vi "clearpath_set_max_speed.vi"(0 "ClearpathComm":T1, 1 "Max Speed":dbl) -> ()   [LabVIEW 2012, in "clearpath_interface.lvlib"]
doc: "Formats a Set Max Speed command (0x210) to change the built-in maximum speed (in m/s). Can not be set to a value greater than the factory default, but can be set lower. Resetting the processor or power cycling the platform will reset the setting to default. Uses the onboard Clearpath library to perform the actual message formatting."
uses:
  clearpath_interface.lvlib
  cwrap_crio.dll
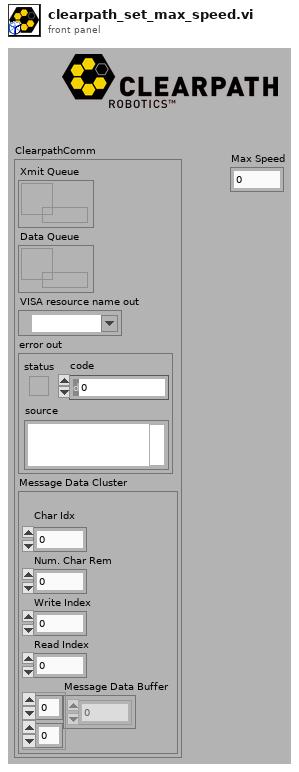
[diagram p1: front panel]
types:
  T1 = cluster{"Xmit Queue":refnum<queue>, "Data Queue":refnum<queue>, "VISA resource name out":refnum<visa-resource-name>, "error out":errorcluster, "Message Data Cluster":cluster{"\nChar Idx":u8, "Num. Char Rem":u8, "Write Index":u8, "Read Index":u8, "Message Data Buffer":u8[][]}}
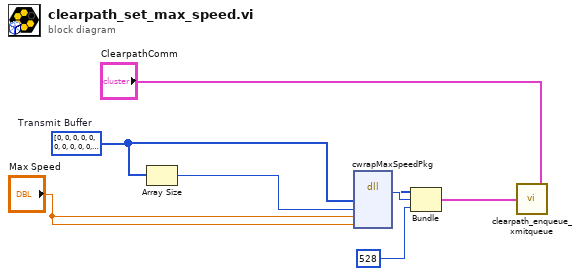
[diagram p0: block diagram]
diagram:
  w5 = u8[] [0, 0, 0, 0, 0, 0, 0, 0, 0, 0, 0, 0, 0, 0, 0, 0, 0, 0, 0, 0, 0, 0, 0, 0, 0, 0, 0, 0, 0, 0, 1, 0, 0, 0, 5]  # Transmit Buffer
  n1 = Array Size(array=w5) -> (size(s)=w6:i32)
  n2 = dll-call lib="C:/Users/tebbeam/Documents/GitHub/IGVC-2013/Code/Project 1.0/Motors/Husky/cwrap_cRIO.*" fn="cwrapMaxSpeedPkg"("buf"=w5, "buf_size"=w6, "max_fwd"="Max Speed", "max_rev"="Max Speed") -> ("return type"=w8:i32, "buf"=w7:u8[])  [unwired: 6 in, 2 out]
  n3 = Bundle("buf"=w7, "return type"=w8, 528) -> (w1:cluster{"buf":u8[], "return type":i32, i32})  [unwired: 1 in]
  n4 = call "clearpath_enqueue_xmitqueue.vi"("ClearpathComm"="ClearpathComm", "Cluster"=w1) -> ()
